vi "Front Panel State.vi"(8 "error in (no error)":errorcluster caption="错误输入（无错误）", 10 "State":T1(ring), 11 "Actor in":refnum<class "RefNums and UICtrl.lvclass">) -> (0 "error out":errorcluster caption="错误输出", 3 "Actor out":refnum<class "RefNums and UICtrl.lvclass">)   [LabVIEW 2020, in "RefNums and UICtrl.lvclass"]
uses:
  RefNums and UICtrl.lvclass
  RefNums and UICtrl.lvclass/RefNums and UICtrl.ctl
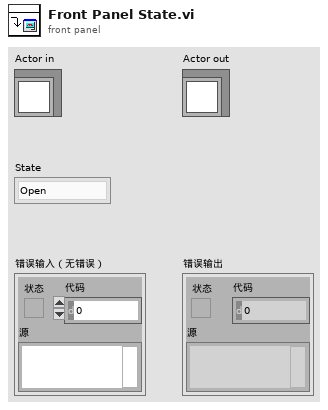
[diagram p1: front panel]
types:
  T1 = enum32{"Open", "Close", "Hide", "Minimize", "Maximize"}
  T2 = enum32{"Invalid", "Standard", "Closed", "Hidden", "Minimized", "Maximized"}
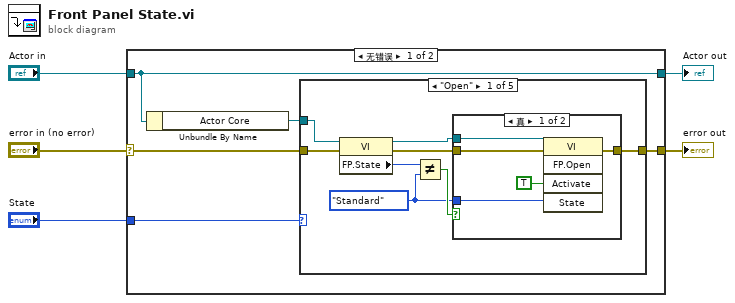
[diagram p0: block diagram]
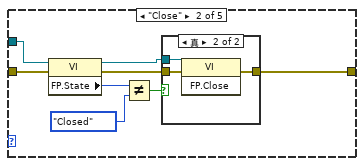
[diagram p3: hidden frame]
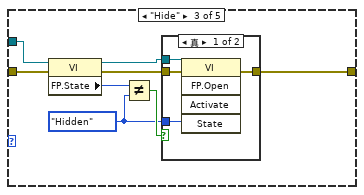
[diagram p5: hidden frame]
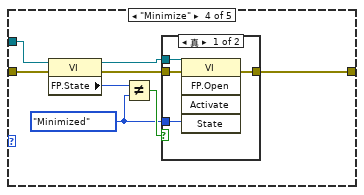
[diagram p7: hidden frame]
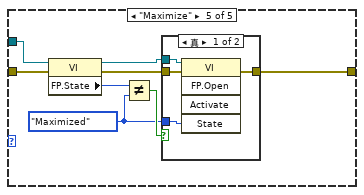
[diagram p9: hidden frame]
diagram:
  n1 = case shown="无错误" "error in (no error)" {
    selector: "error in (no error)" -> [w10 w77]
    tunnel: [w9 w77] -> w4
    tunnel: [w7 w76] -> w2
    tunnel: "Actor in" -> [w7 w76]
    tunnel: "State" -> [w8 _]
    frame No Error {
      n2 = Unbundle By Name(w7) -> ("Actor Core"=w6:refnum<vi>)
      n3 = case shown="\"Open\"" w8 {
        tunnel: w10 -> [w16 w31 w42 w55 w68]
        tunnel: [w18 w32 w44 w57 w70] -> w9
        tunnel: w6 -> [w17 w29 w43 w56 w69]
        frame "Open" {
          w11 = T2."Standard" ("State")
          n4 = property class="VI"(reference=w17, error in=w16) -> (reference out=w14:refnum<vi>, error out=w15:errorcluster, "FP.State"=w13:T2)
          n5 = Not Equal?(x=w13, y=w11) -> (x != y?=w12:bool)
          n6 = case shown="真" w12 {
            tunnel: [w23 w24] -> w18
            tunnel: w15 -> [w22 w24]
            tunnel: w14 -> [w21 _]
            tunnel: w11 -> [w20 _]
            frame True {
              n7 = invoke class="VI" method="FP.Open"(reference=w21, error in=w22, "Activate"=TRUE, "State"=w20) -> (error out=w23:errorcluster)  [unwired: 1 in, 4 out]
            }
            frame False {
            }
          }
        }
        frame "Close" {
          n8 = property class="VI"(reference=w29, error in=w31) -> (reference out=w28:refnum<vi>, error out=w30:errorcluster, "FP.State"=w26:T2)
          n9 = Not Equal?(x=w26, y=T2."Closed" ("Front Panel Window:State")) -> (x != y?=w25:bool)
          n10 = case shown="真" w25 {
            tunnel: [w33 w36] -> w32
            tunnel: w30 -> [w33 w35]
            tunnel: w28 -> [_ w34]
            frame False {
            }
            frame True {
              n11 = invoke class="VI" method="FP.Close"(reference=w34, error in=w35) -> (error out=w36:errorcluster)  [unwired: 1 in, 2 out]
            }
          }
        }
        frame "Hide" {
          w37 = T2."Hidden" ("State")
          n12 = property class="VI"(reference=w43, error in=w42) -> (reference out=w40:refnum<vi>, error out=w41:errorcluster, "FP.State"=w39:T2)
          n13 = Not Equal?(x=w39, y=w37) -> (x != y?=w38:bool)
          n14 = case shown="真" w38 {
            tunnel: [w48 w49] -> w44
            tunnel: w41 -> [w47 w49]
            tunnel: w40 -> [w46 _]
            tunnel: w37 -> [w45 _]
            frame True {
              n15 = invoke class="VI" method="FP.Open"(reference=w46, error in=w47, "State"=w45) -> (error out=w48:errorcluster)  [unwired: 2 in, 4 out]
            }
            frame False {
            }
          }
        }
        frame "Minimize" {
          w50 = T2."Minimized" ("State")
          n16 = property class="VI"(reference=w56, error in=w55) -> (reference out=w53:refnum<vi>, error out=w54:errorcluster, "FP.State"=w52:T2)
          n17 = Not Equal?(x=w52, y=w50) -> (x != y?=w51:bool)
          n18 = case shown="真" w51 {
            tunnel: [w61 w62] -> w57
            tunnel: w54 -> [w60 w62]
            tunnel: w53 -> [w59 _]
            tunnel: w50 -> [w58 _]
            frame True {
              n19 = invoke class="VI" method="FP.Open"(reference=w59, error in=w60, "State"=w58) -> (error out=w61:errorcluster)  [unwired: 2 in, 4 out]
            }
            frame False {
            }
          }
        }
        frame "Maximize" {
          w63 = T2."Maximized" ("State")
          n20 = property class="VI"(reference=w69, error in=w68) -> (reference out=w66:refnum<vi>, error out=w67:errorcluster, "FP.State"=w65:T2)
          n21 = Not Equal?(x=w65, y=w63) -> (x != y?=w64:bool)
          n22 = case shown="真" w64 {
            tunnel: [w74 w75] -> w70
            tunnel: w67 -> [w73 w75]
            tunnel: w66 -> [w72 _]
            tunnel: w63 -> [w71 _]
            frame True {
              n23 = invoke class="VI" method="FP.Open"(reference=w72, error in=w73, "State"=w71) -> (error out=w74:errorcluster)  [unwired: 2 in, 4 out]
            }
            frame False {
            }
          }
        }
      }
    }
    frame Error {
    }
  }
  "error out" <- w4
  "Actor out" <- w2
